vi "helloworld.vi"() -> ()   [LabVIEW 2019]
panel:
  out "String 2":string
  in  "String":string
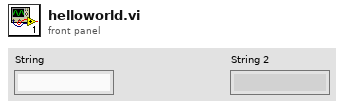
[diagram p1: front panel]
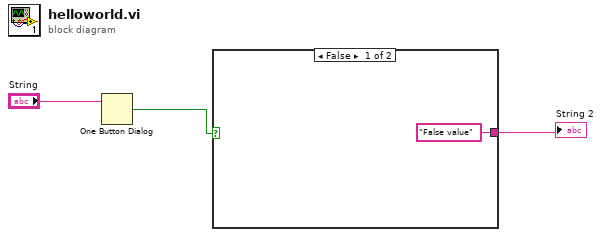
[diagram p0: block diagram]
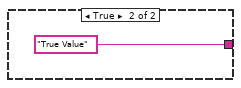
[diagram p2: hidden frame]
diagram:
  n1 = One Button Dialog(message="String") -> (true=w2:bool)  [unwired: 1 in]
  n2 = case shown="False" w2 {
    tunnel: ["False value" ("String 2") "True Value" ("String 2")] -> w1
    frame False {
    }
    frame True {
    }
  }
  "String 2" <- w1
